vi "SetAxisTargetPosition(andForget).vi"(8 "error in (no error)":errorcluster, 10 "AbsolutePosition":i32, 11 "Picomoto8742ControllerClass in":refnum<class "Picomoto8742ControllerClass.lvclass">) -> (0 "error out":errorcluster, 3 "Picomoto8742ControllerClass out":refnum<class "Picomoto8742ControllerClass.lvclass">)   [LabVIEW 2020, in "Picomoto8742ControllerClass.lvclass"]
doc: "Send an absolute move request relative to the active axis, to the physical device"
uses:
  Picomoto8742ControllerClass.lvclass
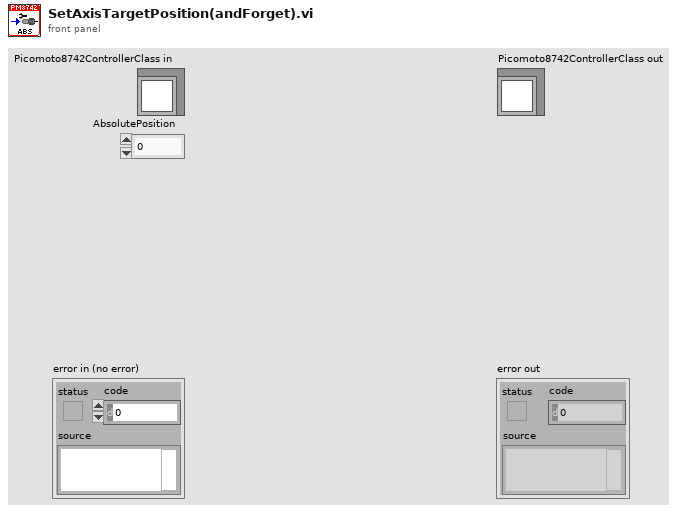
[diagram p1: front panel]
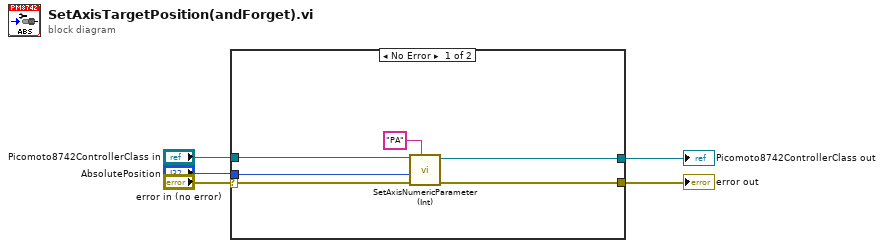
[diagram p0: block diagram]
diagram:
  n1 = case shown="No Error" "error in (no error)" {
    selector: "error in (no error)" -> [w11 w13]
    tunnel: [w7 w13] -> w4
    tunnel: [w6 w12] -> w2
    tunnel: "Picomoto8742ControllerClass in" -> [w9 w12]
    tunnel: "AbsolutePosition" -> [w10 _]
    frame No Error {
      n2 = call "SetAxisNumericParameter(Int).vi"("CMD"="PA" ("string"), "error in (no error)"=w11, "ParameterValue"=w10, "Picomoto8742ControllerClass in"=w9) -> ("error out"=w7:errorcluster, "Picomoto8742ControllerClass Out"=w6:refnum<class "Picomoto8742ControllerClass.lvclass">)  [unwired: 6 in]
    }
    frame Error {
    }
  }
  "error out" <- w4
  "Picomoto8742ControllerClass out" <- w2
